vi "Create Table shell.vi"(0 "Testnames":string[](array[string])) -> (4 "Array":T1[](array[typedef]))   [LabVIEW 2023, in "SQL Database.lvlib"]
uses:
  SQL Database.lvlib
  <vilib>/addons/database/Auxilliary.llb/DB Tools Column Info.ctl
  <vilib>/addons/database/Auxilliary.llb/DB Tools DataTypes.ctl
  <vilib>/addons/database/NI_Database_API.lvlib
panel:
  in  "Is Numeric":bool[](array[boolean])
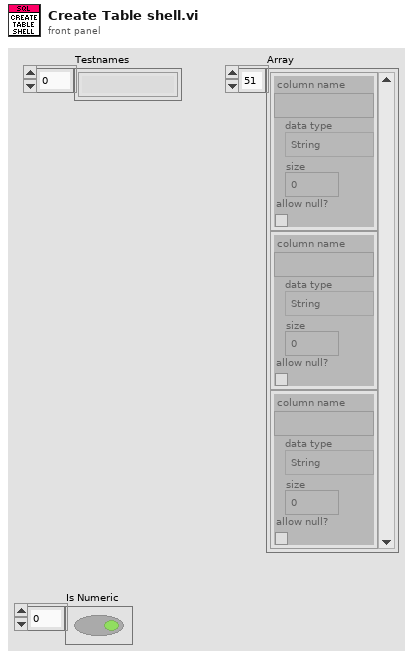
[diagram p1: front panel]
types:
  T1 = typedef "NI_Database_API.lvlib/DB Tools Column Info.ctl" = cluster{"column name":string, "data type":T2, "size":i32, "allow null?":bool}
  T2 = typedef "NI_Database_API.lvlib/DB Tools DataTypes.ctl" = enum16{"String", "Long (I32)", "Single (SGL)", "Double (DBL)", "Date/Time", "Binary"}
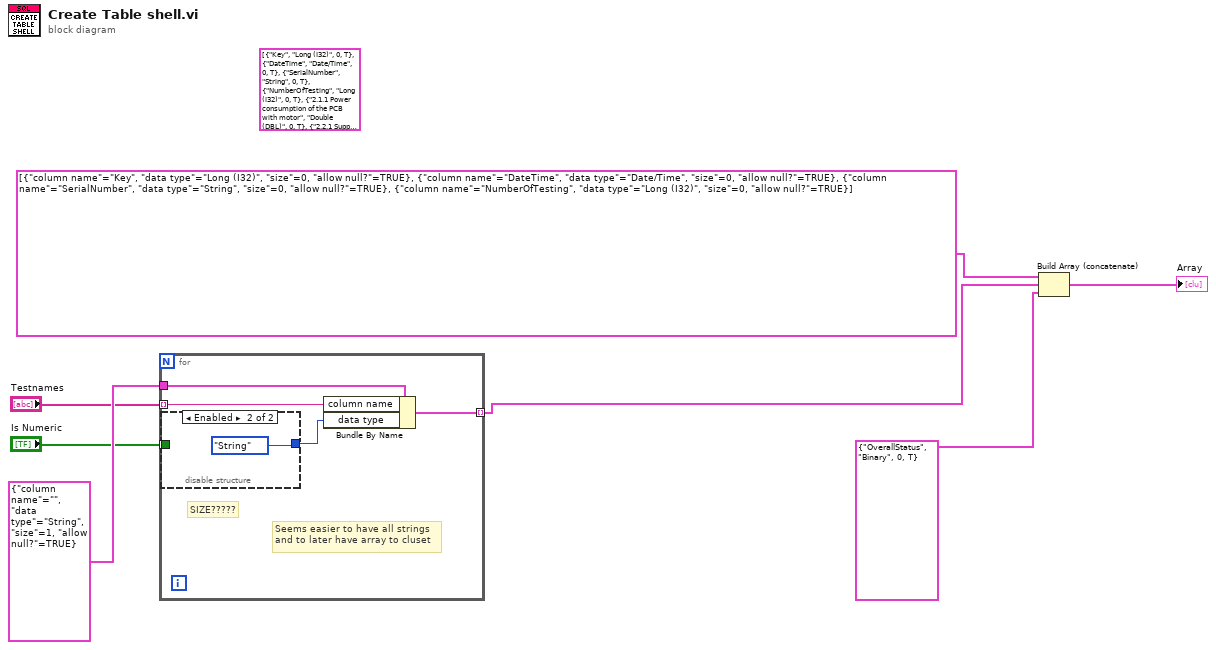
[diagram p0: block diagram]
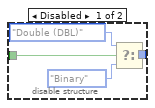
[diagram p2: hidden frame]
diagram:
  (unwired) T1[] [{"column name"="Key", "data type"=enum."Long (I32)", "size"=0, "allow null?"=TRUE}, {"column name"="DateTime", "data type"=enum."Date/Time", "size"=0, "allow null?"=TRUE}, {"column name"="SerialNumber", "data type"=enum."String", "size"=0, "allow null?"=TRUE}, {"column name"="NumberOfTesting", "data type"=enum."Long (I32)", "size"=0, "allow null?"=TRUE}, {"column name"="2.1.1 Power consumption of the PCB with motor", "data type"=enum."Double (DBL)", "size"=0, "allow null?"=TRUE}, {"column name"="2.2.1 Supply Voltage ", "data type"=enum."Binary", "size"=0, "allow null?"=TRUE}, {"column name"="2.2.2 DC Voltage U_MOT TP7", "data type"=enum."Double (DBL)", "size"=0, "allow null?"=TRUE}, {"column name"="2.2.3 DC Voltage LM317 TP8", "data type"=enum."Double (DBL)", "size"=0, "allow null?"=TRUE}, {"column name"="2.2.4 DC Voltage LM25007 TP9", "data type"=enum."Double (DBL)", "size"=0, "allow null?"=TRUE}, {"column name"="2.2.5 DC Voltage NCP01117 TP15", "data type"=enum."Double (DBL)", "size"=0, "allow null?"=TRUE}, {"column name"="3.1.1 Programing", "data type"=enum."Double (DBL)", "size"=0, "allow null?"=TRUE}, {"column name"="4.1.1 Communication Reg 59", "data type"=enum."Double (DBL)", "size"=0, "allow null?"=TRUE}, {"column name"="4.1.2 PCB Identifier Reg", "data type"=enum."Double (DBL)", "size"=0, "allow null?"=TRUE}, {"column name"="4.1.3 Setpoint Reg 0", "data type"=enum."Double (DBL)", "size"=0, "allow null?"=TRUE}, {"column name"="4.1.4.1 Read actual value Reg 21", "data type"=enum."Double (DBL)", "size"=0, "allow null?"=TRUE}, {"column name"="4.1.4.2 Measure Actual value", "data type"=enum."Double (DBL)", "size"=0, "allow null?"=TRUE}, {"column name"="4.1.4.1 Read Stop actual value Reg 21", "data type"=enum."Double (DBL)", "size"=0, "allow null?"=TRUE}, {"column name"="4.1.4.1 Switching On Reg 22", "data type"=enum."Double (DBL)", "size"=0, "allow null?"=TRUE}, {"column name"="4.1.5.2 Measure Switching", "data type"=enum."Double (DBL)", "size"=0, "allow null?"=TRUE}, {"column name"="4.1.4.3 Switching Off Reg 22", "data type"=enum."Binary", "size"=0, "allow null?"=TRUE}, {"column name"="4.1.3.1 Read Positive Half Wave  Reg 1", "data type"=enum."Double (DBL)", "size"=0, "allow null?"=TRUE}, {"column name"="4.1.3.2 Read Negative Half Wave Reg 1", "data type"=enum."Binary", "size"=0, "allow null?"=TRUE}, {"column name"="4.1.3.3 Read Solid Wave Reg 1", "data type"=enum."Binary", "size"=0, "allow null?"=TRUE}, {"column name"="Turn Pot P3 in Middle position", "data type"=enum."Binary", "size"=0, "allow null?"=TRUE}, {"column name"="4.1.7 Feedback potentiometer Reg 8", "data type"=enum."Double (DBL)", "size"=0, "allow null?"=TRUE}, {"column name"="Rotate Encoder G1", "data type"=enum."Binary", "size"=0, "allow null?"=TRUE}, {"column name"="4.1.8 Encoder G1 Reg 13 Read and compare 1", "data type"=enum."Double (DBL)", "size"=0, "allow null?"=TRUE}, {"column name"="4.1.8 Encoder G1 Reg 13 Read and compare 2", "data type"=enum."Double (DBL)", "size"=0, "allow null?"=TRUE}, {"column name"="4.1.9.1 Confirm Turn on DIS1 with Reg 26", "data type"=enum."Binary", "size"=0, "allow null?"=TRUE}, {"column name"="4.1.9.2 Display illuminated", "data type"=enum."Double (DBL)", "size"=0, "allow null?"=TRUE}, {"column name"="4.1.9.3 Confirm Turn off DIS1 with Reg 26", "data type"=enum."Double (DBL)", "size"=0, "allow null?"=TRUE}, {"column name"="4.1.9.4 Confirm Start of Display routine Reg 27", "data type"=enum."Binary", "size"=0, "allow null?"=TRUE}, {"column name"="4.1.9.5 Display test routine", "data type"=enum."Double (DBL)", "size"=0, "allow null?"=TRUE}, {"column name"="4.1.9.6 Confirm Stop of Display routine Reg 27", "data type"=enum."Binary", "size"=0, "allow null?"=TRUE}, {"column name"="4.1.10.1 Confirm Turn on LED D8 Reg 24", "data type"=enum."Double (DBL)", "size"=0, "allow null?"=TRUE}, {"column name"="4.1.10.2 Check if LED turned ON", "data type"=enum."Double (DBL)", "size"=0, "allow null?"=TRUE}, {"column name"="4.1.10.3 Confirm Turn off LED D8 Reg 24", "data type"=enum."Double (DBL)", "size"=0, "allow null?"=TRUE}, {"column name"="4.1.10.4 Check if LED turned Off", "data type"=enum."Double (DBL)", "size"=0, "allow null?"=TRUE}, {"column name"="4.1.11 Motor Voltage Measurement Reg14", "data type"=enum."Binary", "size"=0, "allow null?"=TRUE}, {"column name"="4.1.12.1 Read setting of the engine speed Reg4", "data type"=enum."Double (DBL)", "size"=0, "allow null?"=TRUE}, {"column name"="4.1.12.2 Read Engine running CW Reg3", "data type"=enum."Binary", "size"=0, "allow null?"=TRUE}, {"column name"="4.1.12.3 Read Engine Running status Reg7", "data type"=enum."Binary", "size"=0, "allow null?"=TRUE}, {"column name"="4.1.12.4 Check if Engine is running CW", "data type"=enum."Double (DBL)", "size"=0, "allow null?"=TRUE}, {"column name"="4.1.12.3 Read Hall sensor Running Reg 25 Initial", "data type"=enum."Double (DBL)", "size"=0, "allow null?"=TRUE}, {"column name"="4.1.12.3 Read Hall sensor Running Reg 25 1", "data type"=enum."Binary", "size"=0, "allow null?"=TRUE}, {"column name"="4.1.12.3 Read Hall sensor Running Reg 25 2", "data type"=enum."Double (DBL)", "size"=0, "allow null?"=TRUE}, {"column name"="4.1.12.4 Read Engine stop Reg 3", "data type"=enum."Binary", "size"=0, "allow null?"=TRUE}, {"column name"="4.1.12.5 Read Engine Stop status Reg 7", "data type"=enum."Binary", "size"=0, "allow null?"=TRUE}, {"column name"="4.1.12.5 Check if Engine is running", "data type"=enum."Binary", "size"=0, "allow null?"=TRUE}, {"column name"="4.1.12.6 Read Hall sensor Stop Reg 25 Initial", "data type"=enum."Double (DBL)", "size"=0, "allow null?"=TRUE}, {"column name"="4.1.12.6 Read Hall sensor Stop Reg 25 1", "data type"=enum."Double (DBL)", "size"=0, "allow null?"=TRUE}, {"column name"="4.1.12.6 Read Hall sensor Stop Reg 25 2", "data type"=enum."Double (DBL)", "size"=0, "allow null?"=TRUE}, {"column name"="5.1.1 Read KAT 1 on Reg 1792", "data type"=enum."Double (DBL)", "size"=0, "allow null?"=TRUE}, {"column name"="5.1.2 Serial number write byte ", "data type"=enum."Double (DBL)", "size"=0, "allow null?"=TRUE}, {"column name"="5.1.1 Read KAT 1 close Reg 1794", "data type"=enum."Double (DBL)", "size"=0, "allow null?"=TRUE}, {"column name"="OverallStatus", "data type"=enum."Binary", "size"=0, "allow null?"=TRUE}] ("Array 2")
  n1 = for {
    tunnel: T1 {"column name"="", "data type"=enum."String", "size"=1, "allow null?"=TRUE} ("column information") -> [w12]
    tunnel: "Testnames" -> [w11] mode=indexing
    tunnel: "Is Numeric" -> [w10] mode=indexing
    tunnel: [w8] -> w3 mode=indexing
    # "SIZE?????"
    # "Seems easier to have all strings\nand to later have array to cluset"
    n2 = disable-structure shown="Enabled" {
      disable-tunnel: w10 -> [w16 _]
      disable-tunnel: [w13 DB_Tools_DataTypes."String" ("data type")] -> w9
      frame Disabled {
        n3 = Select(t=DB_Tools_DataTypes."Double (DBL)" ("data type"), s=w16, f=DB_Tools_DataTypes."Binary" ("data type")) -> (s? t:f=w13:T2)
      }
      frame Enabled {
      }
    }
    n4 = Bundle By Name(cluster=w12, "column name"=w11, "data type"=w9) -> (w8:T1)
  }
  n5 = Build Array (concatenate)(T1[] [{"column name"="Key", "data type"=enum."Long (I32)", "size"=0, "allow null?"=TRUE}, {"column name"="DateTime", "data type"=enum."Date/Time", "size"=0, "allow null?"=TRUE}, {"column name"="SerialNumber", "data type"=enum."String", "size"=0, "allow null?"=TRUE}, {"column name"="NumberOfTesting", "data type"=enum."Long (I32)", "size"=0, "allow null?"=TRUE}] ("column information 2"), w3, T1 {"column name"="OverallStatus", "data type"=enum."Binary", "size"=0, "allow null?"=TRUE} ("column information")) -> (→"Array":T1[])
